vi "Read Die Coordinate File.vi"(7 "base path":path=path "C:/Users/er080167/Documents/XP2100/Configuration Files", 11 "FIle_Name":string="XP2100_SH4T die coordinates") -> (3 "Die_Coordinate":string[](array[string]))   [LabVIEW 2013]
uses:
  <vilib>/Utility/file.llb/Read From Spreadsheet File (string).vi
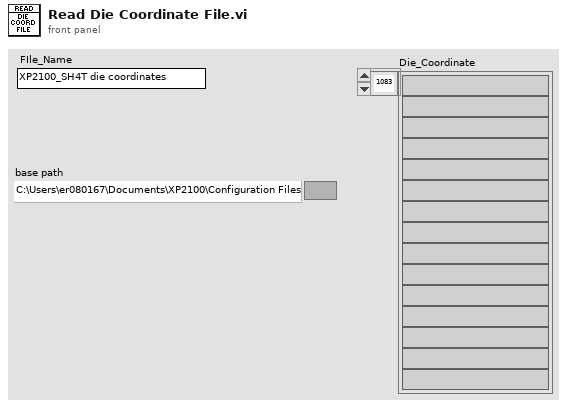
[diagram p1: front panel]
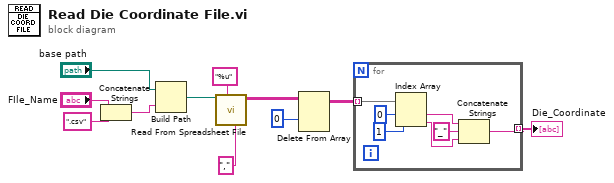
[diagram p0: block diagram]
diagram:
  n1 = Concatenate Strings("FIle_Name", ".csv" ("string")) -> (w9:string)
  n2 = Build Path(base path="base path", name or relative path=w9) -> (appended path=w8:path)
  n3 = call-poly <vilib>:"Read From Spreadsheet File.vi"("delimiter (\\t)"="," ("delimiter (\\t)"), "format (%s)"="%u", "file path (dialog if empty)"=w8) -> ("all rows"=w4:string[][])  [unwired: 4 in, 4 out]
  n4 = Delete From Array(array=w4, index (row)=0) -> (array with subset deleted=w2:string[][])  [unwired: 2 in, 1 out]
  n5 = for {
    tunnel: w2 -> [w16] mode=indexing
    tunnel: [w17] -> w1 mode=indexing
    n6 = Index Array(array=w16, index #1=0 ("index"), index #2=1 ("index")) -> (element #1=w13:string, element #2=w12:string)
    n7 = Concatenate Strings(w13, "_" ("string"), w12) -> (w17:string)
  }
  "Die_Coordinate" <- w1
